vi "Multihead GUI.vi"() -> ()   [LabVIEW 2015, in "Multihead GUI.lvlib"]
uses:
  Multihead GUI Support.llb/Multihead GUI.lvlib
  Multihead GUI Support.llb/Read Termination Message.vi
  Multihead GUI Support.llb/Update Message Routing Info.vi
  Multihead GUI Support.llb/Create Multiple Messages.vi
  Multihead GUI Support.llb/Create Single Message.vi
  Multihead GUI Support.llb/Globals.vi
  Multihead GUI Support.llb/Send Message.vi
  Multihead GUI Support.llb/Main.Constants.vi
  Multihead GUI Support.llb/Queue Registry.vi
  NationalInstruments.VeriStand.ClientAPI
  Multihead GUI Support.llb/AMC.lvlib
  Multihead GUI Support.llb/Single Station Execution.lvlib
  Multihead GUI Support.llb/NI_VS Workspace ExecutionAPI.lvlib
panel:
  in  "NIVS.Gateway IP Address":string="localhost"
  in  "NIVS.Workspace Event":refnum<event-registration>
  in  "Tree":string(tree)
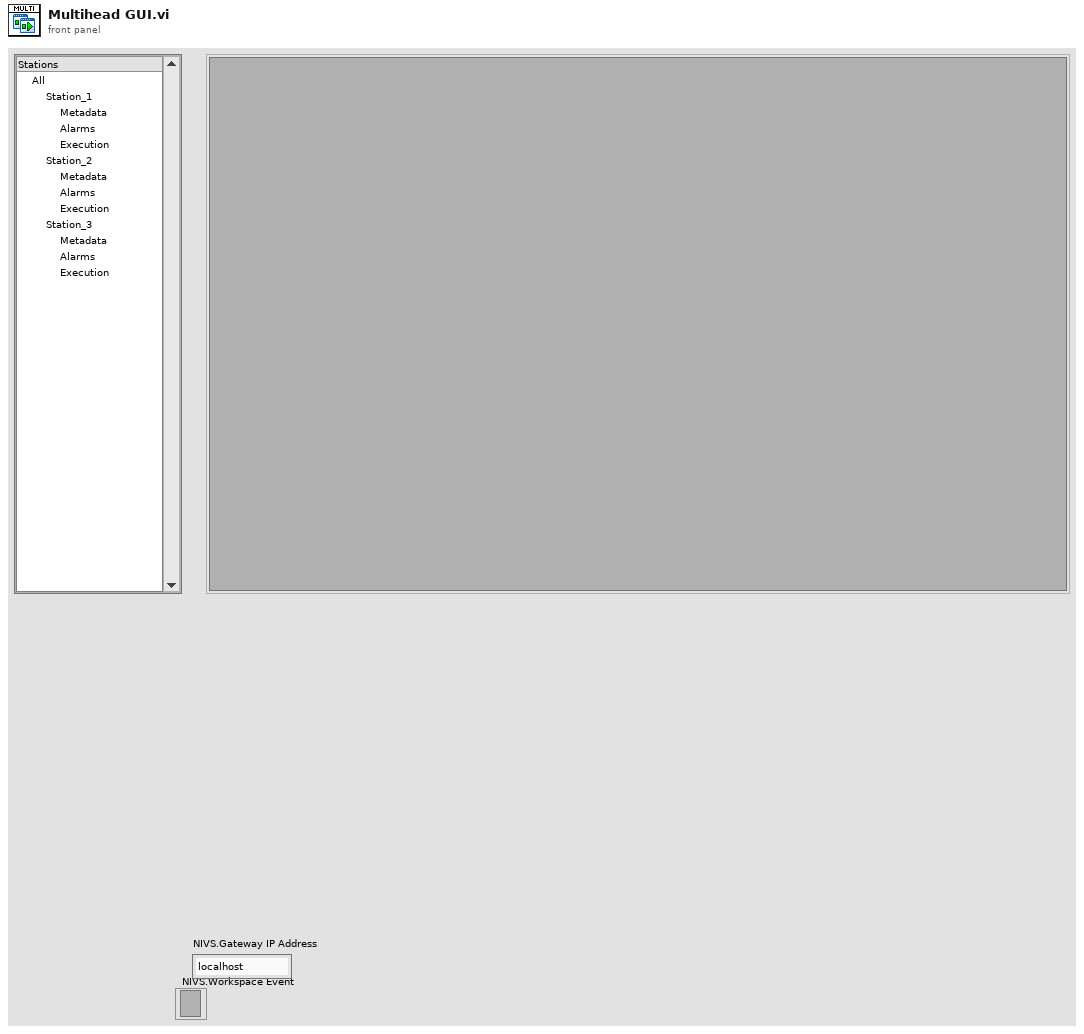
[diagram p1: front panel]
types:
  T1 = cluster{"Station Refs":refnum<vi>[], "NIVS.BaseLogPath":path, "Pages":string[], "NIVS.Gateway IP Address":string, "NIVS.Deployed":bool, "Tree":refnum<vi>, "NIVS.WorkspaceManager":refnum<k24>, "NIVS.SystemStateRefs":cluster{"CustDatRef":refnum<user-event>, "EvtRef":refnum<k27>, "Target State User Event":refnum<user-event>}, "NIVS.Events":cluster{"SystemChangeEvent":refnum<event-registration>, "WorkspaceEvent":refnum<event-registration>}}
  T2 = cluster{"SystemChangeEvent":refnum<event-registration>, "WorkspaceEvent":refnum<event-registration>}
  T3 = cluster{"CustDatRef":refnum<user-event>, "EvtRef":refnum<k27>, "Target State User Event":refnum<user-event>}
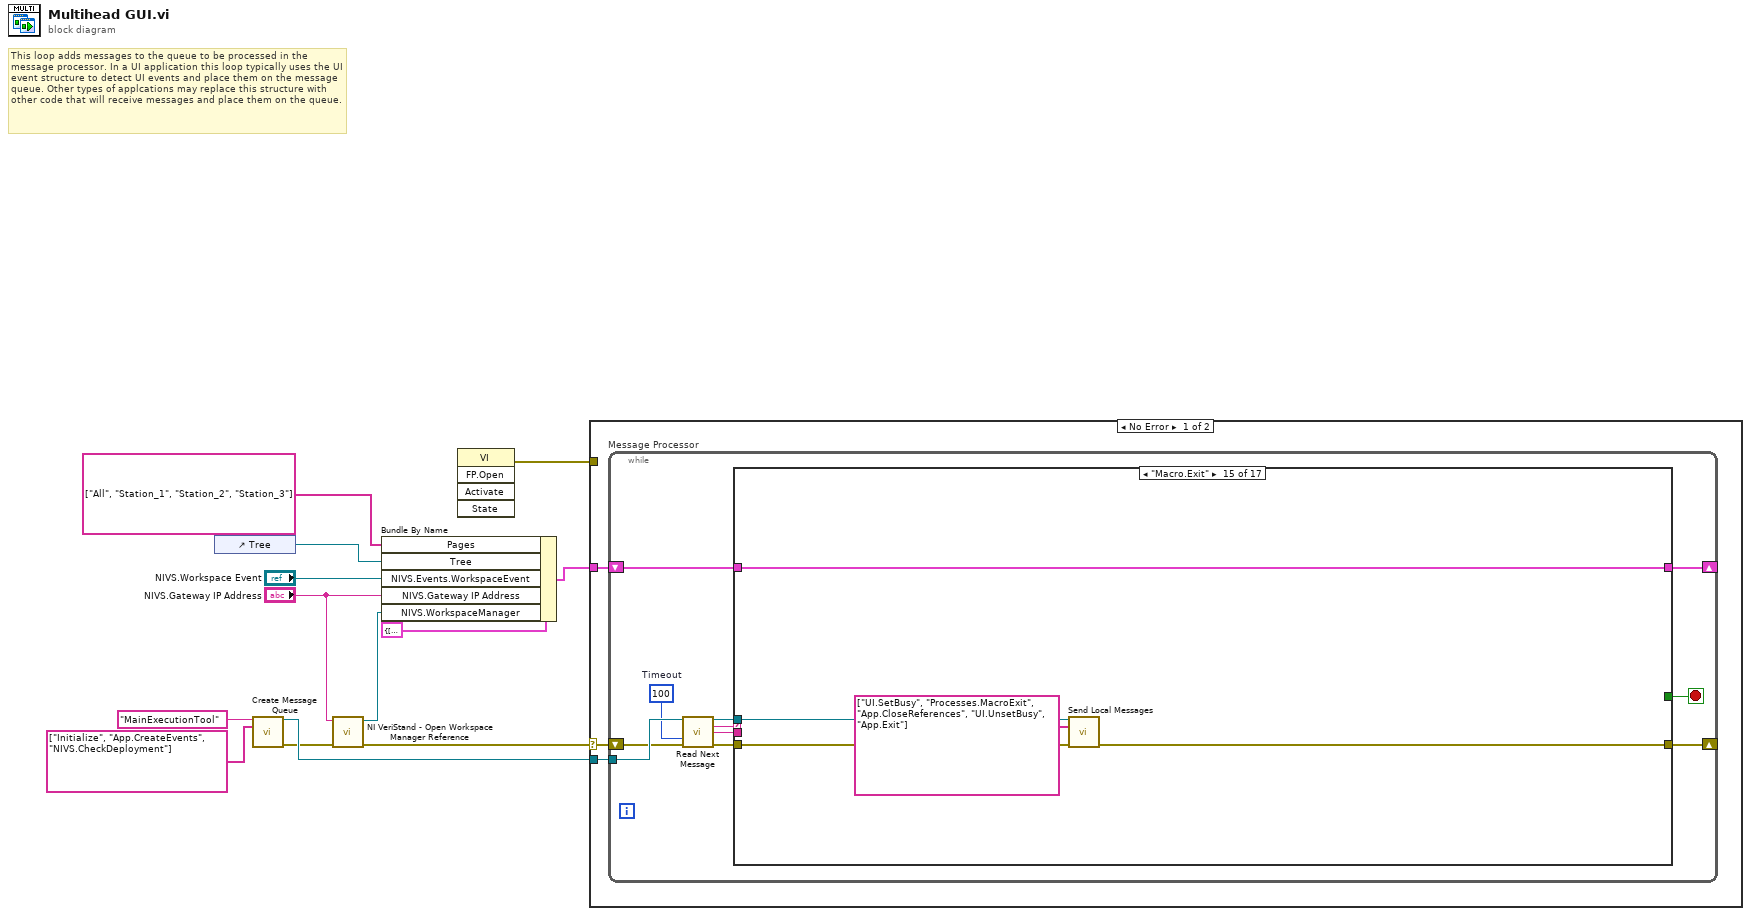
[diagram p0: block diagram]
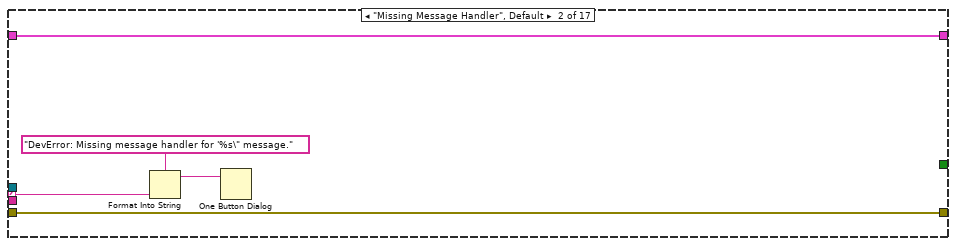
[diagram p3: hidden frame]
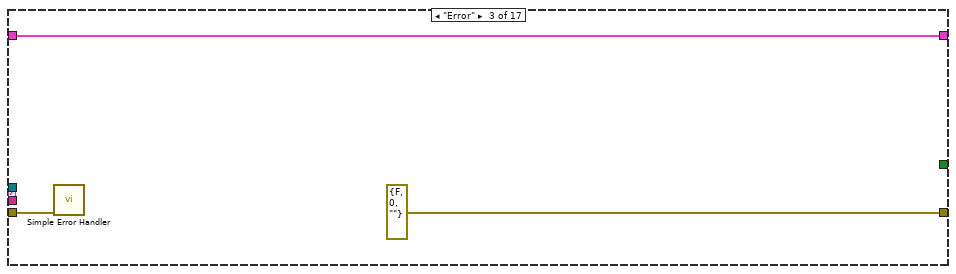
[diagram p4: hidden frame]
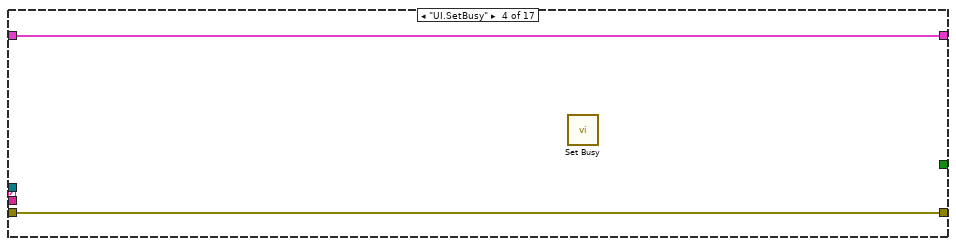
[diagram p5: hidden frame]
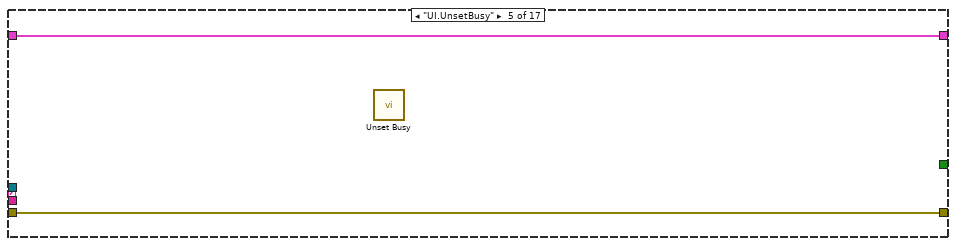
[diagram p6: hidden frame]
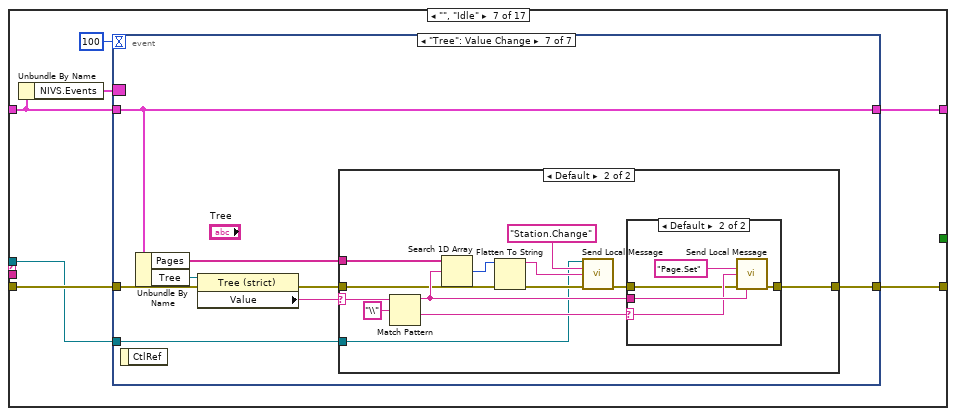
[diagram p8: hidden frame]
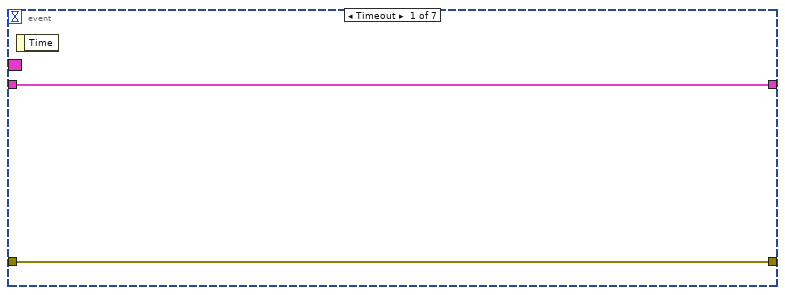
[diagram p9: hidden frame]
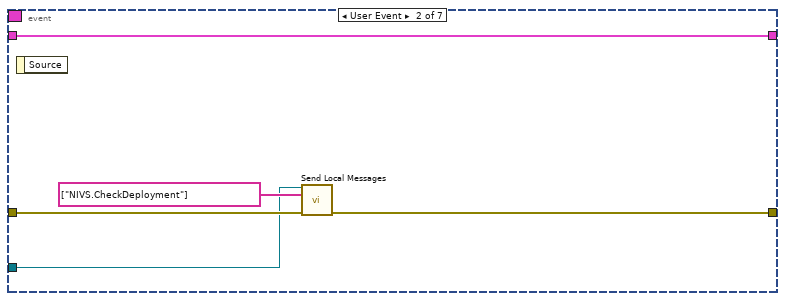
[diagram p10: hidden frame]
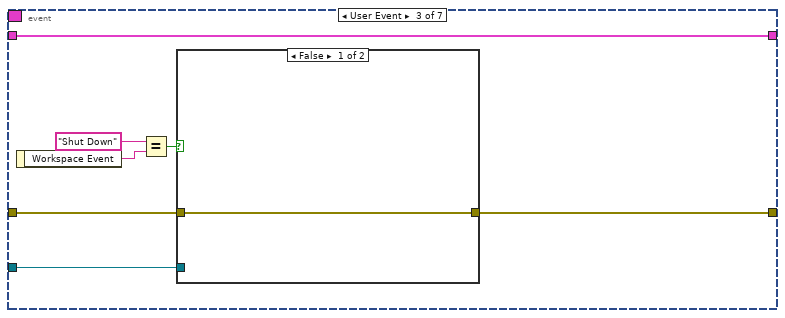
[diagram p11: hidden frame]
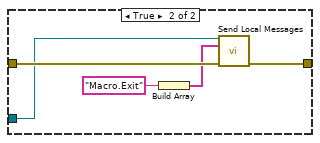
[diagram p12: hidden frame]
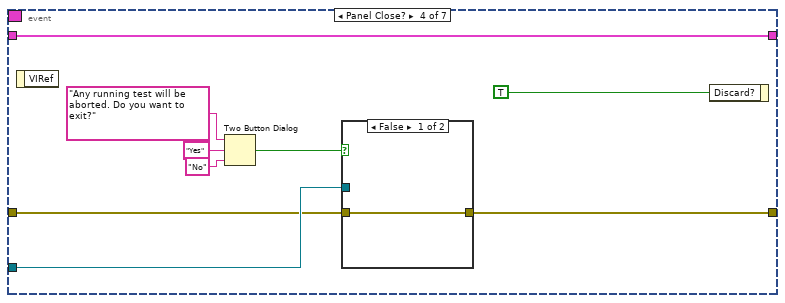
[diagram p13: hidden frame]
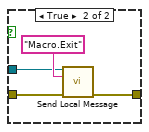
[diagram p14: hidden frame]
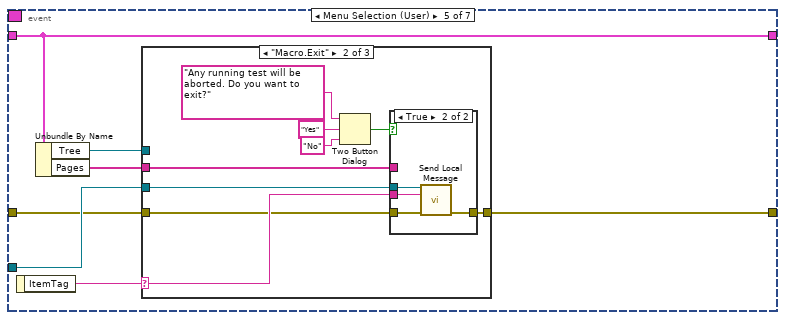
[diagram p15: hidden frame]
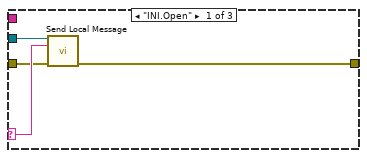
[diagram p16: hidden frame]
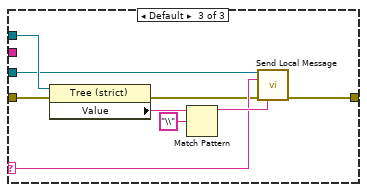
[diagram p18: hidden frame]
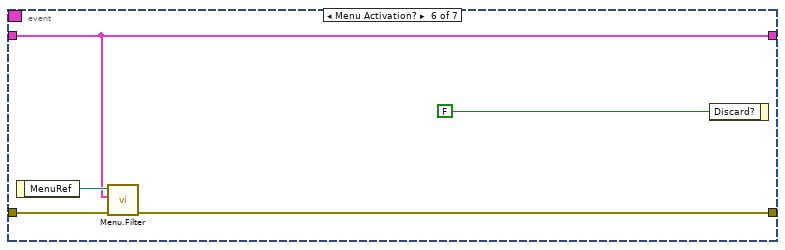
[diagram p19: hidden frame]
diagram:
  # "This loop adds messages to the queue to be processed in the message processor. In a UI application this loop typically uses the UI event structure to detect UI events and place them on the message queue. Other types of applcations may replace this structure with other code that will receive messages and place them on the queue."
  n1 = control-ref of="Tree"() -> (w8:refnum<vi>)
  n2 = call "Create Message Queue.vi"("message queue name"="MainExecutionTool", "initial message names"=string[] ["Initialize", "App.CreateEvents", "NIVS.CheckDeployment"]) -> ("message queue out"=w12:refnum<queue>, "error out"=w5:errorcluster)  [unwired: 12 in]
  n3 = call "NI VeriStand - Open Workspace Manager Reference.vi"("error in (no error)"=w5, "Gateway IP Address (\"\": localhost)"="NIVS.Gateway IP Address") -> ("error out"=w4:errorcluster, "WorkspaceManager"=w3:refnum<k24>)  [unwired: 8 in]
  n4 = Bundle By Name(cluster=T1 {"Station Refs"=[], "NIVS.BaseLogPath"=path "", "Pages"=["All", "Station 1", "Station 2", "Station 3"], "NIVS.Gateway IP Address"="localhost", "NIVS.Deployed"=FALSE, "Tree"=refnum, "NIVS.WorkspaceManager"=refnum, "NIVS.SystemStateRefs"={"CustDatRef"=refnum, "EvtRef"=refnum, "Target State User Event"=refnum}, "NIVS.Events"={"SystemChangeEvent"=refnum, "WorkspaceEvent"=refnum}} ("state variables"), "Pages"=string[] ["All", "Station_1", "Station_2", "Station_3"] ("All Tags"), "Tree"=w8, "NIVS.Events.WorkspaceEvent"="NIVS.Workspace Event", "NIVS.Gateway IP Address"="NIVS.Gateway IP Address", "NIVS.WorkspaceManager"=w3) -> (w7:T1)
  n5 = invoke class="VI" method="FP.Open"() -> (error out=w1:errorcluster)  [unwired: 5 in, 4 out]
  n6 = case shown="No Error" w4 {
    selector: w4 -> [w14 _]
    tunnel: w12 -> [w16 _]
    tunnel: w7 -> [w15 _]
    tunnel: w1 -> [_ _]
    frame No Error {
      n7 = while "Message Processor" {
        shift-left: w14 -> [w22]
        shift-right: [w25] -> _
        tunnel: w16 -> [w23]
        shift-left: w15 -> [w27]
        shift-right: [w26] -> _
        stop <- w17 stop-if-true
        w18 = 100  # Timeout
        n8 = call "Read Next Message.vi"("message queue in"=w23, "timeout (1 ms)"=w18, "error in"=w22) -> ("message queue out"=w24:refnum<queue>, "message name"=w20:string, "message value"=w19:string, "error out"=w21:errorcluster)  [unwired: 5 in, 4 out]
        n9 = case shown="\"Macro.Exit\"" w20 {
          selector: w20 -> [_ w32 _ _ _ _ _ _ _ _ _ _ _ _ _ _ _]
          tunnel: [w29 w34 w37 w39 w41 w43 w49 w154 w156 w163 w178 w190 w202 w215 w236 w238 w255] -> w26
          tunnel: w27 -> [w29 w34 w37 w39 w41 w43 w46 w153 w157 w164 w178 w190 w202 w215 w236 w238 w255]
          tunnel: w24 -> [_ _ _ _ _ _ w47 _ _ _ _ _ _ _ w233 _ w253]
          tunnel: w21 -> [w28 w33 w35 w38 w40 w42 w50 w155 w161 w167 w177 w192 w199 _ w235 w242 w254]
          tunnel: [w28 w33 errorcluster {"status"=FALSE, "code"=0, "source"=""} ("error out") w38 w40 w42 w48 w152 w160 w166 w176 w191 w194 w208 w234 w242 w252] -> w25
          tunnel: w19 -> [_ _ _ _ _ _ _ _ _ _ _ w193 w200 _ _ _ _]
          tunnel: [_ _ _ _ _ _ _ _ _ _ _ _ _ _ _ _ TRUE] -> w17
          frame "---------- Framework Operations ----------" {
            # "Dummy case to add a seperator in the Case Structure menu"
          }
          frame "Missing Message Handler", Default {
            n10 = Format Into String(format string="DevError: Missing message handler for '%s\" message." ("message"), w32) -> (resulting string=w30:string)  [unwired: 2 in, 1 out]
            n11 = One Button Dialog(message=w30) -> ()  [unwired: 2 out]
          }
          frame "Error" {
            n12 = call "Simple Error Handler.vi"("error in (no error)"=w35) -> ()  [unwired: 1 in, 8 out]
          }
          frame "UI.SetBusy" {
            n13 = call "Set Busy.vi"() -> ()  [unwired: 10 in, 2 out]
          }
          frame "UI.UnsetBusy" {
            n14 = call "Unset Busy.vi"() -> ()  [unwired: 11 in, 1 out]
          }
          frame "---------- Application Operations ----------" {
            # "Dummy case to add a seperator in the Case Structure menu"
          }
          frame "", "Idle" {
            n15 = Unbundle By Name(w46) -> ("NIVS.Events"=w45:T2)
            n16 = event shown="[6] \"Tree\": Value Change" {
              selector: w45 -> [_ _ _ _ _ _ _]
              dyn-events: _ -> [_ _ _ _ _ _ _]
              timeout: 100 -> [_ _ _ _ _ _ _]
              tunnel: w50 -> [w51 w57 w61 w77 w87 w121 w131]
              tunnel: w46 -> [w52 w53 w59 w79 w89 w119 w125]
              tunnel: [w52 w53 w59 w79 w89 w119 w125] -> w49
              tunnel: [w51 w54 w58 w76 w86 w120 w128] -> w48
              tunnel: w47 -> [_ w55 w60 w78 w90 _ w126]
              event Timeout {
                n17 = event-data() -> ()  [unwired: 2 out]
              }
              event User Event {
                n18 = event-data() -> ()  [unwired: 2 out]
                n19 = call "Send Local Messages.vi"("message queue in"=w55, "message names"=string[] ["NIVS.CheckDeployment"], "error in"=w57) -> ("error out"=w54:errorcluster)  [unwired: 10 in, 2 out]
              }
              event User Event {
                n20 = event-data() -> ("Workspace Event"=w63:string)  [unwired: 1 out]
                n21 = Equal?(x="Shut Down" ("y"), y=w63) -> (x = y?=w62:bool)
                n22 = case shown="False" w62 {
                  tunnel: w61 -> [w65 w70]
                  tunnel: [w65 w69] -> w58
                  tunnel: w60 -> [_ w66]
                  frame False {
                  }
                  frame True {
                    n23 = Build Array("Macro.Exit" ("y")) -> (w68:string[])
                    n24 = call "Send Local Messages.vi"("message queue in"=w66, "message names"=w68, "error in"=w70) -> ("error out"=w69:errorcluster)  [unwired: 10 in, 2 out]
                  }
                }
              }
              event Panel Close? {
                n25 = event-data() -> ()  [unwired: 2 out]
                n26 = Two Button Dialog(message="Any running test will be aborted. Do you want to exit?", 1:"No" ("F button name (\"Cancel\")"), 2:"Yes" ("T button name (\"OK\")")) -> (T button?=w71:bool)
                n27 = case shown="False" w71 {
                  tunnel: w78 -> [_ w83]
                  tunnel: w77 -> [w80 w82]
                  tunnel: [w80 w81] -> w76
                  frame False {
                  }
                  frame True {
                    n28 = call "Send Local Message.vi"("message queue in"=w83, "message name"="Macro.Exit", "error in"=w82) -> ("error out"=w81:errorcluster)  [unwired: 10 in, 2 out]
                  }
                }
                n29 = event-data("Discard?"=TRUE) -> ()  [unwired: 1 in, 1 out]
              }
              event Menu Selection (User) {
                n30 = event-data() -> ("ItemTag"=w91:string)  [unwired: 1 out]
                n31 = Unbundle By Name(w89) -> ("Tree"=w88:refnum<vi>, "Pages"=w85:string[])
                n32 = case shown="\"Macro.Exit\"" w91 {
                  selector: w91 -> [w94 w103 w114]
                  tunnel: w88 -> [_ _ w115]
                  tunnel: w90 -> [w95 w104 w110]
                  tunnel: w87 -> [w93 w102 w113]
                  tunnel: [w92 w101 w111] -> w86
                  tunnel: w85 -> [_ w96 _]
                  frame "INI.Open" {
                    n33 = call "Send Local Message.vi"("message queue in"=w95, "message name"=w94, "error in"=w93) -> ("error out"=w92:errorcluster)  [unwired: 10 in, 2 out]
                  }
                  frame "Macro.Exit" {
                    n34 = Two Button Dialog(message="Any running test will be aborted. Do you want to exit?", 1:"No" ("F button name (\"Cancel\")"), 2:"Yes" ("T button name (\"OK\")")) -> (T button?=w97:bool)
                    n35 = case shown="True" w97 {
                      tunnel: w104 -> [_ w109]
                      tunnel: w103 -> [_ w107]
                      tunnel: w102 -> [w105 w108]
                      tunnel: [w105 w106] -> w101
                      tunnel: w96 -> [_ _]
                      frame False {
                      }
                      frame True {
                        n36 = call "Send Local Message.vi"("message queue in"=w109, "message name"=w107, "error in"=w108) -> ("error out"=w106:errorcluster)  [unwired: 10 in, 2 out]
                      }
                    }
                  }
                  frame Default {
                    n37 = property class="Tree (strict)"(reference=w115, error in=w113) -> (error out=w112:errorcluster, "Value"=w118:string)  [unwired: 1 out]
                    n38 = Match Pattern(string=w118, regular expression="\\") -> (before substring=w116:string)  [unwired: 1 in, 3 out]
                    n39 = call "Send Local Message.vi"("message queue in"=w110, "receiver process (\"\" - local)"=w116, "message name"=w114, "error in"=w112) -> ("error out"=w111:errorcluster)  [unwired: 9 in, 2 out]
                  }
                }
              }
              event Menu Activation? {
                n40 = event-data() -> ("MenuRef"=w122:refnum<k9>)  [unwired: 1 out]
                n41 = call "Menu.Filter.vi"("error in (no error)"=w121, "state variables in"=w119, "Menu in"=w122) -> ("error out"=w120:errorcluster)  [unwired: 8 in]
                n42 = event-data("Discard?"=FALSE) -> ()  [unwired: 1 in, 1 out]
              }
              event "Tree": Value Change {
                n43 = event-data() -> ()  [unwired: 2 out]
                n44 = Unbundle By Name(w125) -> ("Pages"=w127:string[], "Tree"=w130:refnum<vi>)
                n45 = property class="Tree (strict)"(reference=w130, error in=w131) -> (error out=w129:errorcluster, "Value"=w124:string)  [unwired: 1 out]
                n46 = case shown="Default" w124 {
                  selector: w124 -> [_ w133]
                  tunnel: w129 -> [w132 w139]
                  tunnel: [w132 w136] -> w128
                  tunnel: w127 -> [_ w135]
                  tunnel: w126 -> [_ w134]
                  frame "" {
                  }
                  frame Default {
                    n47 = Match Pattern(string=w133, regular expression="\\") -> (before substring=w140:string, after substring=w141:string)  [unwired: 1 in, 2 out]
                    n48 = Search 1D Array(1D array=w135, element=w140) -> (index of element=w143:i32)  [unwired: 1 in]
                    n49 = Flatten To String(anything=w143, error in (no error)=w139) -> (data string=w142:string, error out=w138:errorcluster)  [unwired: 2 in, 1 out]
                    n50 = call "Send Local Message.vi"("message queue in"=w134, "message name"="Station.Change", "message value"=w142, "error in"=w138) -> ("error out"=w137:errorcluster)  [unwired: 9 in, 2 out]
                    n51 = case shown="Default" w141 {
                      selector: w141 -> [_ w150]
                      tunnel: w140 -> [_ w151]
                      tunnel: w137 -> [w146 w148]
                      tunnel: [w146 w147] -> w136
                      frame "" {
                      }
                      frame Default {
                        n52 = call "Send Local Message.vi"("receiver process (\"\" - local)"=w151, "message name"="Page.Set", "message value"=w150, "error in"=w148) -> ("error out"=w147:errorcluster)  [unwired: 9 in, 2 out]
                      }
                    }
                  }
                }
              }
            }
          }
          frame "Initialize" {
            n53 = call "VI.Launch.vi"("error in (no error)"=w155, "state variables in"=w153) -> ("error out"=w152:errorcluster, "state variables out"=w154:T1)  [unwired: 8 in]
          }
          frame "App.CreateEvents" {
            n54 = Unbundle By Name(w157) -> ("NIVS.WorkspaceManager"=w162:refnum<k24>)
            n55 = call "NI VeriStand - Open Engine State Change Notification.vi"("error in (no error)"=w161, "WorkspaceManager in"=w162) -> ("error out"=w160:errorcluster, "SystemStateRefs"=w159:T3, "SystemChangeEventRef"=w158:refnum<event-registration>)  [unwired: 6 in, 1 out]
            n56 = Bundle By Name(cluster=w157, "NIVS.Events.SystemChangeEvent"=w158, "NIVS.SystemStateRefs"=w159) -> (w156:T1)
          }
          frame "NIVS.CheckDeployment" {
            n57 = Unbundle By Name(w164) -> ("NIVS.WorkspaceManager"=w165:refnum<k24>)
            n58 = call "NI VeriStand - Get System State.vi"("error in (no error)"=w167, "WorkspaceManager in"=w165) -> ("error out"=w166:errorcluster, "System State"=w168:u8)  [unwired: 5 in, 3 out]
            n59 = case shown="1" w168 {
              tunnel: w164 -> [w171 w174]
              tunnel: [w170 w172] -> w163
              frame 0, Default {
                # "Not connected"
                n60 = Bundle By Name(cluster=w171, "NIVS.Deployed"=FALSE ("Connected")) -> (w170:T1)
              }
              frame 1 {
                # "Connected"
                n61 = Bundle By Name(cluster=w174, "NIVS.Deployed"=TRUE ("Connected")) -> (w172:T1)
              }
            }
          }
          frame "INI.Open" {
            n62 = Unbundle By Name(w178) -> ("NIVS.Events.WorkspaceEvent"=w183:refnum<event-registration>)
            n63 = Not A Number/Path/Refnum?(number/path/refnum=w183) -> (NaN/Path/Refnum?=w184:bool)
            n64 = case shown="False" w184 {
              tunnel: [w186 w188] -> w182
              frame False {
                n65 = property class="VI"() -> ("Path"=w187:path)  [unwired: 2 in, 2 out]
                n66 = Strip Path(path=w187) -> (stripped path=w186:path)  [unwired: 1 out]
              }
              frame True {
                n67 = call "Application Directory.vi"() -> ("Application Directory"=w188:path)
              }
            }
            n68 = global read "Main.Constants.vi" "INI.FileName"() -> (w185:string)
            n69 = Build Path(base path=w182, name or relative path=w185) -> (appended path=w181:path)
            n70 = Path To String(path=w181) -> (string=w175:string)
            n71 = Concatenate Strings("explorer " ("string"), w175) -> (w179:string)
            n72 = call "System Exec.vi"("error in (no error)"=w177, "command line"=w179) -> ("error out"=w176:errorcluster)  [unwired: 6 in, 3 out]
          }
          frame "Page.Published" {
            n73 = Unbundle By Name(w190) -> ("Tree"=w189:refnum<vi>)
            n74 = property class="Tree (strict)"(reference=w189, error in=w192, "Value"=w193) -> (error out=w191:errorcluster)  [unwired: 1 out]
          }
          frame "Station.Change" {
            n75 = Unflatten From String(type=0 ("x-1"), binary string=w200, error in (no error)=w199) -> (value=w197:i32, error out=w195:errorcluster)  [unwired: 2 in, 1 out]
            n76 = Unbundle By Name(w202) -> ("Station Refs"=w201:refnum<vi>[])
            n77 = Index Array(array=w201, index=w197) -> (element=w196:refnum<vi>)
            n78 = invoke on="Sub Panel" class="SubPnl" method="Insert VI"(error in=w195, "VI Ref"=w196) -> (error out=w194:errorcluster)  [unwired: 2 in, 3 out]
          }
          frame "Processes.MacroExit" {
            w205 = 50
            w212 = "Macro.Exit"
            n79 = Unbundle By Name(w215) -> ("Pages"=w214:string[])
            n80 = Delete From Array(array=w214, index=0) -> (deleted portion=w213:string, array with subset deleted=w204:string[])  [unwired: 1 in]
            n81 = call "Send Local Message.vi"("receiver process (\"\" - local)"=w213, "message name"=w212) -> ("error out"=w211:errorcluster)  [unwired: 11 in, 2 out]
            n82 = for {
              N: w205 -> [_]
              tunnel: w213 -> [w231]
              tunnel: w211 -> [w229]
              tunnel: [w228] -> w210
              stop <- w228 stop-if-true
              n83 = call "Get Queue From Registry.vi"("name"=w231, "error in"=w229) -> ("error out"=w228:errorcluster)  [unwired: 12 in, 1 out]
              n84 = Wait Until Next ms Multiple(millisecond multiple=u32 100) -> ()  [unwired: 1 out]
            }
            n85 = call "Clear Errors.vi"("error in (no error)"=w210) -> ("error out"=w209:errorcluster)  [unwired: 5 in, 1 out]
            n86 = for {
              tunnel: w204 -> [w225] mode=indexing
              tunnel: w212 -> [w226]
              tunnel: w209 -> [w227]
              tunnel: [w224] -> w206
              n87 = call "Send Local Message.vi"("receiver process (\"\" - local)"=w225, "message name"=w226, "error in"=w227) -> ("error out"=w224:errorcluster)  [unwired: 10 in, 2 out]
            }
            n88 = for {
              tunnel: w206 -> [w219]
              tunnel: w205 -> [w218]
              tunnel: w204 -> [w217] mode=indexing
              tunnel: [w216] -> w203
              n89 = for {
                N: w218 -> [_]
                tunnel: w217 -> [w223]
                tunnel: [w221] -> w216
                tunnel: w219 -> [w220]
                stop <- w221 stop-if-true
                n90 = call "Get Queue From Registry.vi"("name"=w223, "error in"=w220) -> ("error out"=w221:errorcluster)  [unwired: 12 in, 1 out]
                n91 = Wait Until Next ms Multiple(millisecond multiple=u32 100) -> ()  [unwired: 1 out]
              }
            }
            n92 = call "Clear Errors.vi"("error in (no error)"=w203) -> ("error out"=w208:errorcluster)  [unwired: 5 in, 1 out]
          }
          frame "Macro.Exit" {
            n93 = call "Send Local Messages.vi"("message queue in"=w233, "message names"=string[] ["UI.SetBusy", "Processes.MacroExit", "App.CloseReferences", "UI.UnsetBusy", "App.Exit"], "error in"=w235) -> ("error out"=w234:errorcluster)  [unwired: 10 in, 2 out]
          }
          frame "App.CloseReferences" {
            n94 = Unbundle By Name(w238) -> ("Station Refs"=w237:refnum<vi>[], "NIVS.Events"=w241:T2, "NIVS.SystemStateRefs"=w240:T3, "NIVS.WorkspaceManager"=w239:refnum<k24>)
            n95 = flat-sequence {
              tunnel: w241 -> [w250]
              tunnel: w240 -> [w249]
              tunnel: w239 -> [w248]
              tunnel: w237 -> [w247]
              tunnel: [w246] -> _
              tunnel: [w245] -> _
              tunnel: [w244] -> _
              tunnel: [w243] -> _
              frame #0 {
                n96 = call "NI VeriStand - Close Workspace Manager Reference.vi"("WorkspaceManager"=w248) -> ("error out"=w243:errorcluster)  [unwired: 10 in]
                n97 = call "NI VeriStand - Close Engine State Change Notification.vi"("SystemStateRefs"=w249) -> ("error out"=w244:errorcluster)  [unwired: 10 in]
                n98 = Unregister For Events(event registration refnum=w250) -> (error out=w245:errorcluster)  [unwired: 1 in]
                n99 = Close Reference(reference=w247) -> (error out=w246:errorcluster)  [unwired: 1 in]
              }
            }
          }
          frame "App.Exit" {
            # "Destroy message queue >> this will halt the UI event handler loop"
            # "Stop the VI\n>> Perform any cleanup tasks in this message case.\n>> Clear display before closing."
            n100 = call "Destroy Message Queue.vi"("message queue in"=w253, "error in"=w254) -> ("error out"=w252:errorcluster)  [unwired: 11 in, 2 out]
            n101 = invoke class="VI" method="FP.Close"() -> ()  [unwired: 3 in, 3 out]
          }
        }
      }
    }
    frame Error {
      n102 = One Button Dialog(message="NI VeriStand is not open. Please open NI VeriStand before running this utility.") -> (true=w256:bool)  [unwired: 1 in]
      n103 = flat-sequence {
        tunnel: w256 -> [_]
        frame #0 {
          n104 = disable-structure shown="Enabled" {
            disable-tunnel: [w258 _] -> _
            frame Enabled {
              n105 = invoke class="VI" method="FP.Close"() -> (error out=w258:errorcluster)  [unwired: 3 in, 2 out]
            }
            frame Disabled {
            }
          }
        }
      }
    }
  }
